vi "Find Item In Library.vi"(10 "Label.Text":string, 11 "LVClassLibrary in":refnum<vi>) -> (2 "Found":bool, 3 "ProjectItem Ref":refnum<vi>)   [LabVIEW 2018, in "DVR Accessor Library.lvlib"]
uses:
  DVR Accessor Library.lvlib
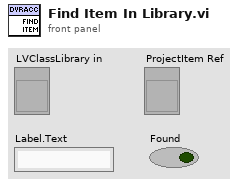
[diagram p1: front panel]
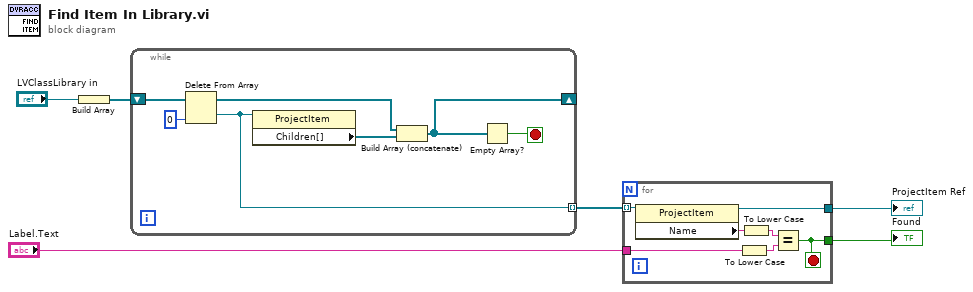
[diagram p0: block diagram]
diagram:
  n1 = Build Array("LVClassLibrary in") -> (w2:refnum<vi>[])
  n2 = while {
    shift-right: [w8] -> _
    shift-left: w2 -> [w13]
    tunnel: [w9] -> w1 mode=indexing
    stop <- w7 stop-if-true
    n3 = Delete From Array(array=w13, index=0) -> (deleted portion=w9:refnum<vi>, array with subset deleted=w11:refnum<vi>[])  [unwired: 1 in]
    n4 = property class="ProjectItem"(reference=w9) -> ("Children[]"=w12:refnum<vi>[])  [unwired: 1 in, 2 out]
    n5 = Build Array (concatenate)(w11, w12) -> (w8:refnum<vi>[])
    n6 = Empty Array?(array=w8) -> (empty?=w7:bool)
  }
  n7 = for {
    tunnel: w1 -> [w20] mode=indexing
    tunnel: "Label.Text" -> [w17]
    tunnel: [w16] -> w6
    tunnel: [w15] -> w5
    stop <- w15 stop-if-true
    n8 = property class="ProjectItem"(reference=w20) -> (reference out=w16:refnum<vi>, "Name"=w19:string)  [unwired: 1 in, 1 out]
    n9 = To Lower Case(string=w17) -> (all lower case string=w18:string)
    n10 = To Lower Case(string=w19) -> (all lower case string=w14:string)
    n11 = Equal?(x=w14, y=w18) -> (x = y?=w15:bool)
  }
  "ProjectItem Ref" <- w6
  "Found" <- w5
